vi "Replace Message Template Control.vi"(8 "error in (no error)":errorcluster, 10 "Class Path":path, 11 "App Inst":refnum<vi>) -> (0 "error out":errorcluster)   [LabVIEW 2020, in "Message Rescripter.lvlib"]
uses:
  Message Rescripter.lvlib
  MessageMakerProvider/_Message Maker/Message Maker.lvlib
  <vilib>/Utility/traverseref.llb/TRef TravTarget.ctl
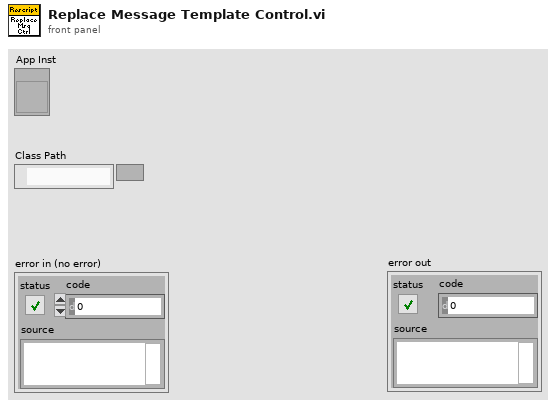
[diagram p1: front panel]
types:
  T1 = typedef "TRef TravTarget.ctl" = enum16{"FP", "BD", "Other"}
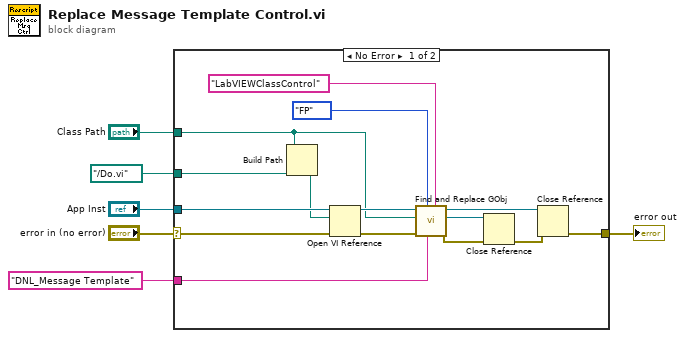
[diagram p0: block diagram]
diagram:
  n1 = case shown="No Error" "error in (no error)" {
    selector: "error in (no error)" -> [w10 w22]
    tunnel: "App Inst" -> [w21 _]
    tunnel: [w12 w22] -> w5
    tunnel: "Class Path" -> [w9 _]
    tunnel: path "../Do.vi" ("Relative Path to Method") -> [w8 _]
    tunnel: "DNL_Message Template" ("Class Control Label") -> [w7 _]
    frame No Error {
      n2 = Build Path(base path=w9, name or relative path=w8) -> (appended path=w11:path)
      n3 = Open VI Reference(application reference (local)=w21, vi path=w11, error in (no error)=w10) -> (vi reference=w20:refnum<vi>, error out=w19:errorcluster)  [unwired: 3 in]
      n4 = call "Find and Replace GObj.vi"("GObj Class Name"="LabVIEWClassControl" ("Class Name"), "GObj Label"=w7, "Traverse Target"=TRef_TravTarget."FP", "error in (no error)"=w19, "Class Path"=w9, "vi reference in"=w20) -> ("error out"=w15:errorcluster, "Replace"=w13:refnum<vi>, "vi reference out"=w16:refnum<vi>)  [unwired: 3 in]
      n5 = Close Reference(reference=w13, error in (no error)=w15) -> (error out=w14:errorcluster)
      n6 = Close Reference(reference=w16, error in (no error)=w14) -> (error out=w12:errorcluster)
    }
    frame Error {
    }
  }
  "error out" <- w5
